vi "Write Rules Parser Parameters.vi"(9 "Parameters":string, 11 "CDependencyInspection in":refnum<class "CDependencyInspection.lvclass">) -> (3 "CDependencyInspection out":refnum<class "CDependencyInspection.lvclass">)   [LabVIEW 2020, in "DependencyInspection.lvlib" / "CDependencyInspection.lvclass"]
uses:
  CDependencyInspection.lvclass
  CDependencyInspection.lvclass/CDependencyInspection.ctl
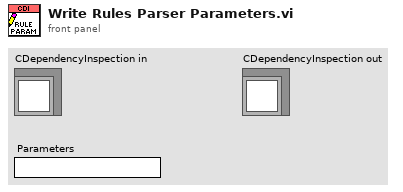
[diagram p1: front panel]
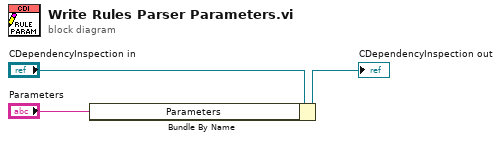
[diagram p0: block diagram]
diagram:
  n1 = Bundle By Name(cluster="CDependencyInspection in", "Parameters"="Parameters") -> (→"CDependencyInspection out":refnum<class "CDependencyInspection.lvclass">)
